vi "IntegrateFRF.vi"(8 "delay (sec)":dbl, 9 "Output":u16(ring)=1 items=["Accelerometer", "Accel (speed)", "Microphone", "Vibrometer"], 11 "Complex FRF":cluster{"t0":dbl, "dt":dbl, "Y":cdb[]}) -> (2 "Complex FRF out":cluster{"t0":dbl, "dt":dbl, "Y":cdb[]}, 3 "FRF out":cluster{"t0":dbl, "dt":dbl, dbl[]}(graph)={"t0"=0.0, "dt"=1.0, array[24001 elements]})   [LabVIEW 2022 SP3]
panel:
  in  "Tab Control 2":enum32{"Page 1", "Page 2"}(tab)
  out "change in real term":cluster{"t0":dbl, "dt":dbl, "Y":dbl[]}[](graph)
  in  "Tab Control":enum32{"Page 1", "Page 2", "Page 3", "Page 4"}(tab)
  out "Magnitude FRF":cluster{"t0":dbl, "dt":dbl, dbl[]}(graph)={"t0"=0.0, "dt"=1.0, array[24001 elements]}
  out "Integral FRF":cluster{"t0":dbl, "dt":dbl, dbl[]}(graph)={"t0"=0.0, "dt"=1.0, array[24001 elements]}
  out "change in mag":cluster{"t0":dbl, "dt":dbl, dbl[]}[](graph)
  out "change in phase":cluster{"t0":dbl, "dt":dbl, dbl[]}[](graph)
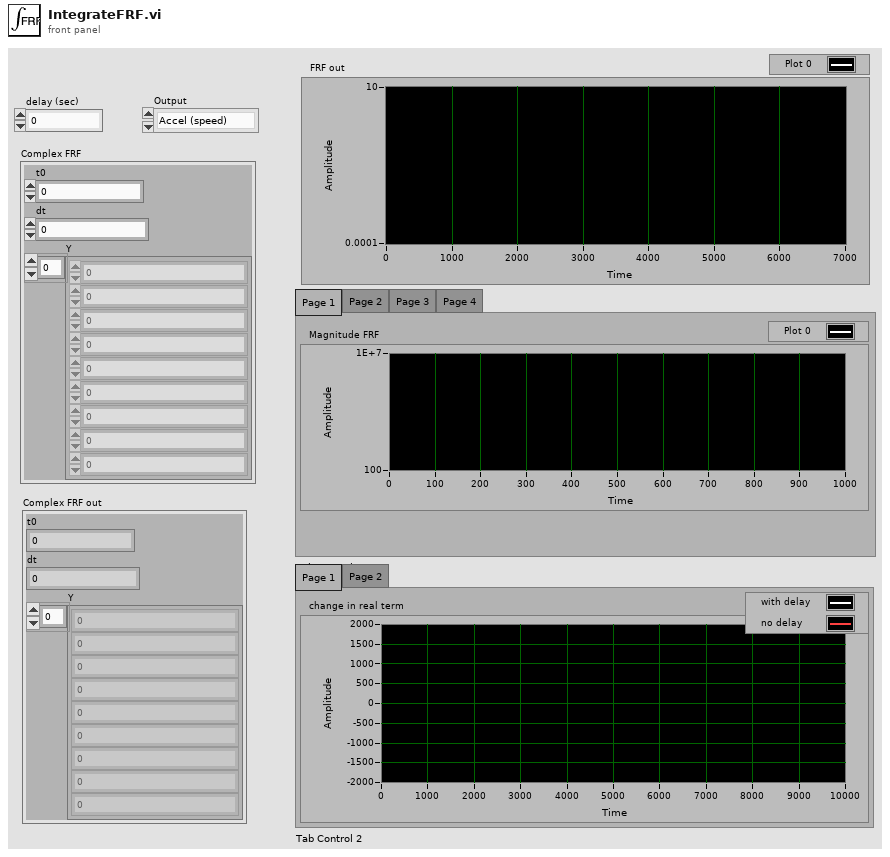
[diagram p1: front panel]
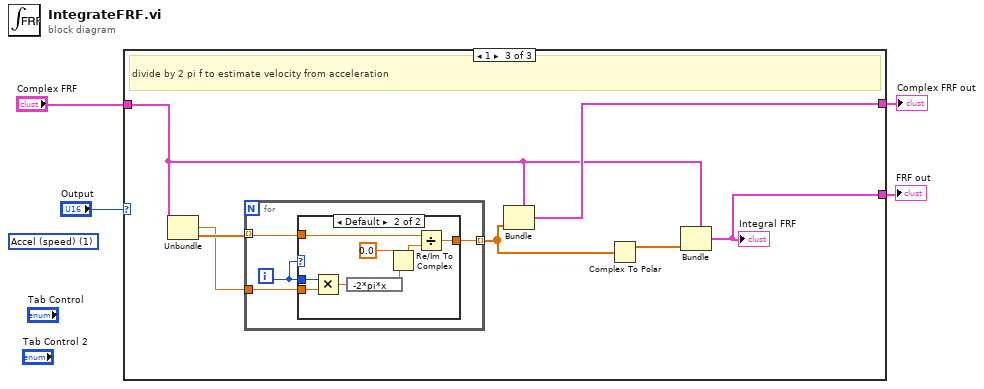
[diagram p0: block diagram]
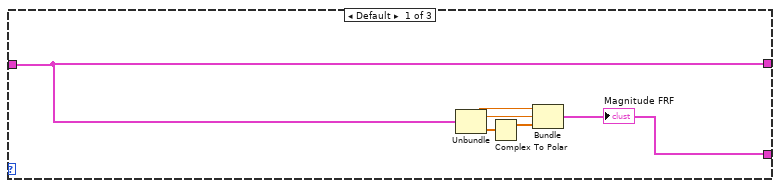
[diagram p2: hidden frame]
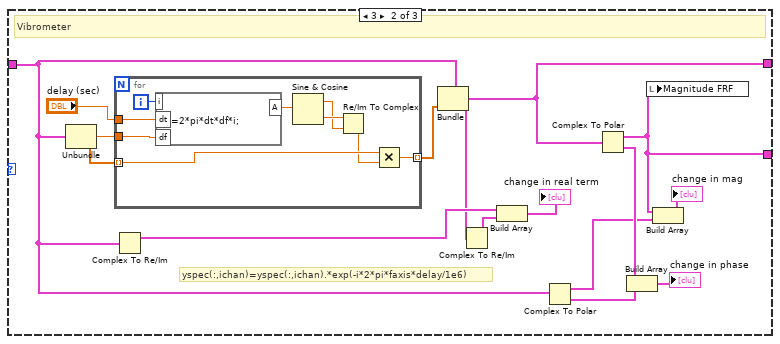
[diagram p3: hidden frame]
diagram:
  (unwired) u16 1 items=["Accelerometer", "Accel (speed)", "Microphone", "Vibrometer"] ("Output")
  n1 = case shown="1" "Output" {
    tunnel: [w5 w16 w36] -> w4
    tunnel: [w6 w11 w37] -> w3
    tunnel: "Complex FRF" -> [w6 w12 w35]
    frame Default {
      n2 = Unbundle(w6) -> ("t0"=w8:dbl, "dt"=w7:dbl, "Y"=w9:cdb[])
      n3 = Complex To Polar(r * e^(i*theta)=w9) -> (r=w10:dbl[])  [unwired: 1 out]
      n4 = Bundle("t0"=w8, "dt"=w7, w10) -> (w5:cluster{"t0":dbl, "dt":dbl, dbl[]})  [unwired: 1 in]
      "Magnitude FRF" <- w5
    }
    frame 3 {
      # "yspec(:,ichan)=yspec(:,ichan).*exp(-i*2*pi*faxis*delay/1e6)"
      # "Vibrometer"
      n5 = Unbundle(w12) -> ("dt"=w25:dbl, "Y"=w20:cdb[])  [unwired: 1 out]
      n6 = for {
        tunnel: w25 -> [w33]
        tunnel: "delay (sec)" -> [w31]
        tunnel: w20 -> [w30] mode=indexing
        tunnel: [w34] -> w17 mode=indexing
        i -> [w32]
        n7 = formula code="A=2*pi*dt*df*i;"("i"=w32, "df"=w33, "dt"=w31) -> ("A"=w29:dbl)
        n8 = Sine & Cosine(0:w29) -> (1:w27:dbl, 2:w28:dbl)
        n9 = Re/Im To Complex(1:w27, 2:w28) -> (0:w26:cdb)
        n10 = Multiply(x=w30, y=w26) -> (x*y=w34:cdb)
      }
      n11 = Complex To Re/Im(x + iy=w12) -> (x=w23:cluster{"t0":dbl, "dt":dbl, "Y":dbl[]})  [unwired: 1 out]
      n12 = Bundle(cluster=w12, "Y"=w17) -> (w11:cluster{"t0":dbl, "dt":dbl, "Y":cdb[]})  [unwired: 2 in]
      n13 = Complex To Re/Im(x + iy=w11) -> (x=w22:cluster{"t0":dbl, "dt":dbl, "Y":dbl[]})  [unwired: 1 out]
      n14 = Build Array(w23, w22) -> (→"change in real term":cluster{"t0":dbl, "dt":dbl, "Y":dbl[]}[])
      n15 = Complex To Polar(r * e^(i*theta)=w12) -> (r=w14:cluster{"t0":dbl, "dt":dbl, "Y":dbl[]}, theta=w13:cluster{"t0":dbl, "dt":dbl, "Y":dbl[]})
      n16 = Complex To Polar(r * e^(i*theta)=w11) -> (r=w16:cluster{"t0":dbl, "dt":dbl, "Y":dbl[]}, theta=w15:cluster{"t0":dbl, "dt":dbl, "Y":dbl[]})
      n17 = Build Array(w15, w13) -> (→"change in phase":cluster{"t0":dbl, "dt":dbl, "Y":dbl[]}[])
      n18 = local write "Magnitude FRF"(w16) -> ()
      n19 = Build Array(w16, w14) -> (→"change in mag":cluster{"t0":dbl, "dt":dbl, "Y":dbl[]}[])
    }
    frame 1 {
      # "divide by 2 pi f to estimate velocity from acceleration"
      n20 = Unbundle(w35) -> ("dt"=w39:dbl, "Y"=w40:cdb[])  [unwired: 1 out]
      n21 = for {
        tunnel: w40 -> [w44] mode=indexing
        tunnel: w39 -> [w45]
        tunnel: [w43] -> w38 mode=indexing
        i -> [w42]
        n22 = case shown="Default" w42 {
          tunnel: w45 -> [_ w53]
          tunnel: w42 -> [_ w52]
          tunnel: w44 -> [w46 w49]
          tunnel: [w46 w48] -> w43
          frame 0 {
          }
          frame Default {
            n23 = Multiply(x=w52, y=w53) -> (x*y=w51:dbl)
            n24 = expression code="-2*pi*x"(w51) -> (w47:dbl)
            n25 = Re/Im To Complex(1:w47, 2:0.0 ("x")) -> (0:w50:cdb)
            n26 = Divide(x=w49, y=w50) -> (x/y=w48:cdb)
          }
        }
      }
      n27 = Bundle(cluster=w35, "Y"=w38) -> (w37:cluster{"t0":dbl, "dt":dbl, "Y":cdb[]})  [unwired: 2 in]
      n28 = Complex To Polar(r * e^(i*theta)=w38) -> (r=w41:dbl[])  [unwired: 1 out]
      n29 = Bundle(cluster=w35, "Y"=w41) -> (w36:cluster{"t0":dbl, "dt":dbl, "Y":cdb[]})  [unwired: 2 in]
      "Integral FRF" <- w36
    }
  }
  "FRF out" <- w4
  "Complex FRF out" <- w3
